vi "Validate Name.vi"(8 "error in (no error)":errorcluster, 10 "Name In":string, 11 "Process In":refnum<class "Process.lvclass">) -> (0 "error out":errorcluster, 2 "Name Out":string, 3 "Process Out":refnum<class "Process.lvclass">)   [LabVIEW 2020, in "Process.lvclass"]
uses:
  Process.lvclass
  <vilib>/Utility/error.llb/Error Cluster From Error Code.vi
  <vilib>/ErrorRing/Error Ring.xnode
  Process.lvclass/Process.ctl
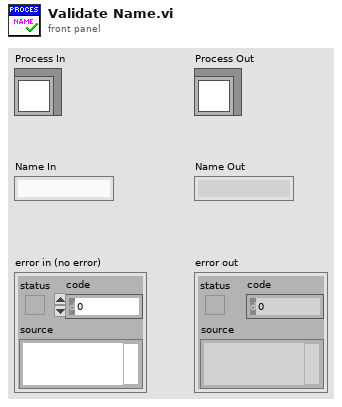
[diagram p1: front panel]
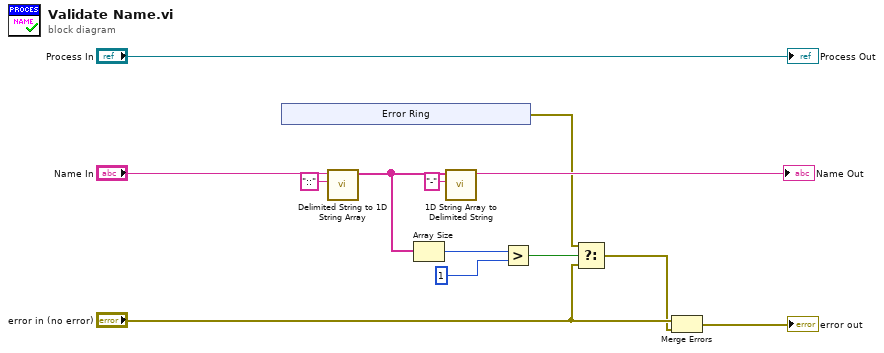
[diagram p0: block diagram]
diagram:
  n1 = xnode "Error Ring"() -> ("error out"=w1:errorcluster)
  n2 = call <vilib>:"Delimited String to 1D String Array.vi"("delimiter"="::", "delimited string"="Name In") -> ("string array"=w8:string[])  [unwired: 9 in]
  n3 = Array Size(array=w8) -> (size(s)=w7:i32)
  n4 = call <vilib>:"1D String Array to Delimited String.vi"("delimiter"="-", "string array"=w8) -> ("delimited string"=→"Name Out":string)  [unwired: 9 in]
  n5 = Greater?(x=w7, y=1) -> (0:w5:bool)
  n6 = Select(t=w1, s=w5, f="error in (no error)") -> (s? t:f=w2:errorcluster)
  n7 = Merge Errors("error in (no error)", w2) -> (→"error out":errorcluster)
  "Process Out" <- "Process In"
